vi "Set Magnet Field.vi"(4 "Axis":T1, 6 "Mode":T2, 8 "error in (no error)":errorcluster, 9 "Target Rate (T/min)":dbl, 10 "Target Field (T)":dbl, 11 "IPS120 in":refnum<class "IPS120.lvclass">) -> (0 "error out":errorcluster, 3 "IPS120 out":refnum<class "IPS120.lvclass">)   [LabVIEW 2016, in "IPS120.lvclass"]
uses:
  IPS120.lvclass
  <userlib>/LevyLab/Levylab Instruments/Instrument Types/Cryostat/Typedefs/Magnet Mode--Enum.ctl
  <userlib>/LevyLab/Levylab Instruments/Instrument Types/Cryostat/Typedefs/Magnet Axis--Enum.ctl
  API/Typedefs/Targets - Cluster.ctl
  API/IPS-120-API.lvlib
  IPS-120.lvlib
  <userlib>/LevyLab/Levylab Instruments/Instrument Types/Cryostat/Instrument.Cryostat.lvclass
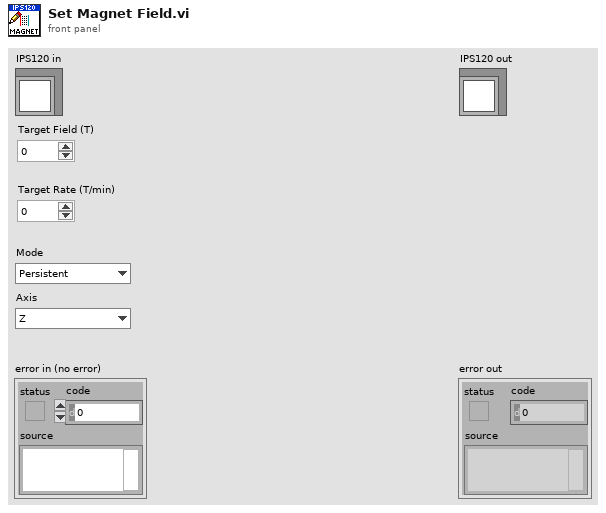
[diagram p1: front panel]
types:
  T1 = typedef "Instrument.Cryostat.lvclass/Magnet Axis--Enum.ctl" = enum16{"Z", "X", "Y"}
  T2 = typedef "Instrument.Cryostat.lvclass/Magnet Mode--Enum.ctl" = enum16{"Persistent", "Driven"}
  T3 = typedef "IPS-120.lvlib/Targets - Cluster.ctl" = cluster{"Target Field (T)":dbl, "Target Field Rate (T/min)":dbl}
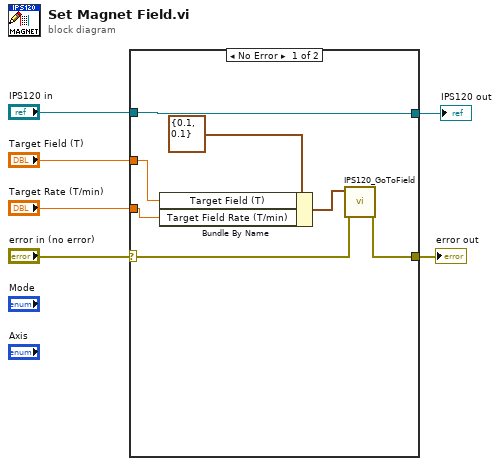
[diagram p0: block diagram]
diagram:
  n1 = case shown="No Error" "error in (no error)" {
    selector: "error in (no error)" -> [w13 w15]
    tunnel: [w12 w15] -> w5
    tunnel: "Target Field (T)" -> [w10 _]
    tunnel: "Target Rate (T/min)" -> [w9 _]
    tunnel: "IPS120 in" -> [w7 w14]
    tunnel: [w7 w14] -> w1
    frame No Error {
      n2 = Bundle By Name(cluster=T3 {"Target Field (T)"=0.1, "Target Field Rate (T/min)"=0.1} ("IPS120 Targets"), "Target Field (T)"=w10, "Target Field Rate (T/min)"=w9) -> (w8:T3)
      n3 = call "IPS120_GoToField.vi"("error in"=w13, "IPS120 Targets"=w8) -> ("error out"=w12:errorcluster)  [unwired: 9 in]
    }
    frame Error {
    }
  }
  "error out" <- w5
  "IPS120 out" <- w1
